vi "界面UI.vi"() -> ()   [LabVIEW 2016, in "德润超标留样.lvlib"]
uses:
  <vilib>/Utility/miscctls.llb/LVPointTypeDef.ctl
  <vilib>/Utility/config.llb/NI_LVConfig.lvlib
panel:
  in  "时间等比采样":u16=10
  in  "单次采样量":u16=500
  in  "修改门禁密码":bool
  in  "远程复位":bool
  in  "排空当前瓶":bool
  in  "采样方式":enum16{"单采", "双重"}(ring)
  in  "远程留样":bool
  in  "选择留样瓶":bool
  in  "排空留样瓶":bool
  out "采样器状态":T1
  out "Registers":u16[](array[numeric])
  in  "打开串口":bool
  in  "释放串口":bool
  in  "留样模式":T2(ring)=enum."外控留样"
  in  "采样启动":bool
  in  "停止命令":bool
  in  "切换采样器状态":bool
  in  "时间校准":bool
  out "source":string
  out "通讯":bool
  # "只在待机时启动有效"
  # "只在停止时切换有效"
  # "只在待机时启动有效"
  # "只在待机时切换有效"
  # "只在待机时启动有效"
  # "默认：500ml（5-1000）ml （只在停止时写有效）"
  # "默认：10min（2-9999）min （只在停止时写有效）"
  # "德润DR803L超标留样"
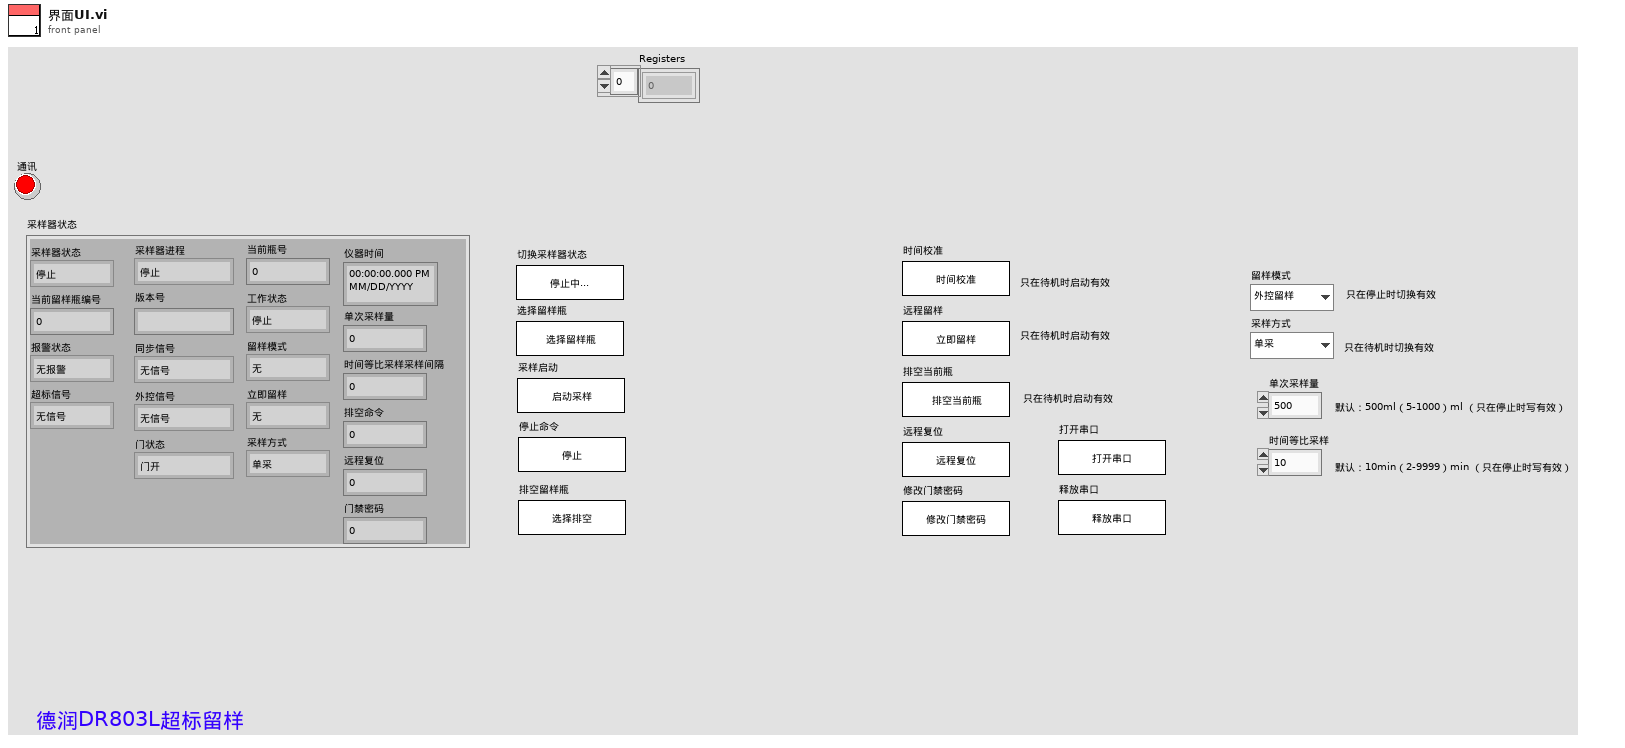
[diagram p1: front panel]
types:
  T1 = cluster{"采样器状态":enum16{"停止", "运行"}, "当前留样瓶编号":u16, "报警状态":enum16{"无报警", "缺水报警"}, "超标信号":enum16{"无信号", "超标信号"}, "采样器进程":enum16{"停止", "待机", "定位校正", "移除瓶盖", "采样瓶排空", "管路润洗", "管存", "进样", "瓶盖密封", "管路排空", "调整采样位置", "采样结束", "采样瓶润洗", "瓶润洗排空"}, "版本号":string, "同步信号":enum16{"无信号", "同步信号"}, "外控信号":enum16{"无信号", "外控信号"}, "门状态":enum16{"门开", "门关"}, "当前瓶号":u16, "工作状态":enum16{"停止", "采样中"}, "留样模式":enum16{"无", "定时留样", "时间等比例", "超标留样", "同步留样", "外控留样"}, "立即留样":enum16{"无", "远程留样"}, "采样方式":enum16{"单采", "双重"}, "仪器时间":timestamp, "单次采样量":u16, "时间等比采样采样间隔":u16, "排空命令":u16, "远程复位":u16, "门禁密码":u16}
  T2 = enum16{"", "定时留样", "时间等比", "超标留样", "同步留样", "外控留样"}
  T3 = typedef "LVPointTypeDef.ctl" = cluster{"Horizontal":i16, "Vertical":i16}
  T4 = typedef "NI_LVConfig.lvlib/Config Data RefNum.ctl" = refnum<k1>
  T5 = typedef "LVDateTimeRec.ctl" = cluster{"秒数的小数部分":dbl, "秒":i32, "分":i32, "时":i32, "日":i32, "月":i32, "年":i32, "天数（周）":i32, "天数（年）":i32, "DST":i32}
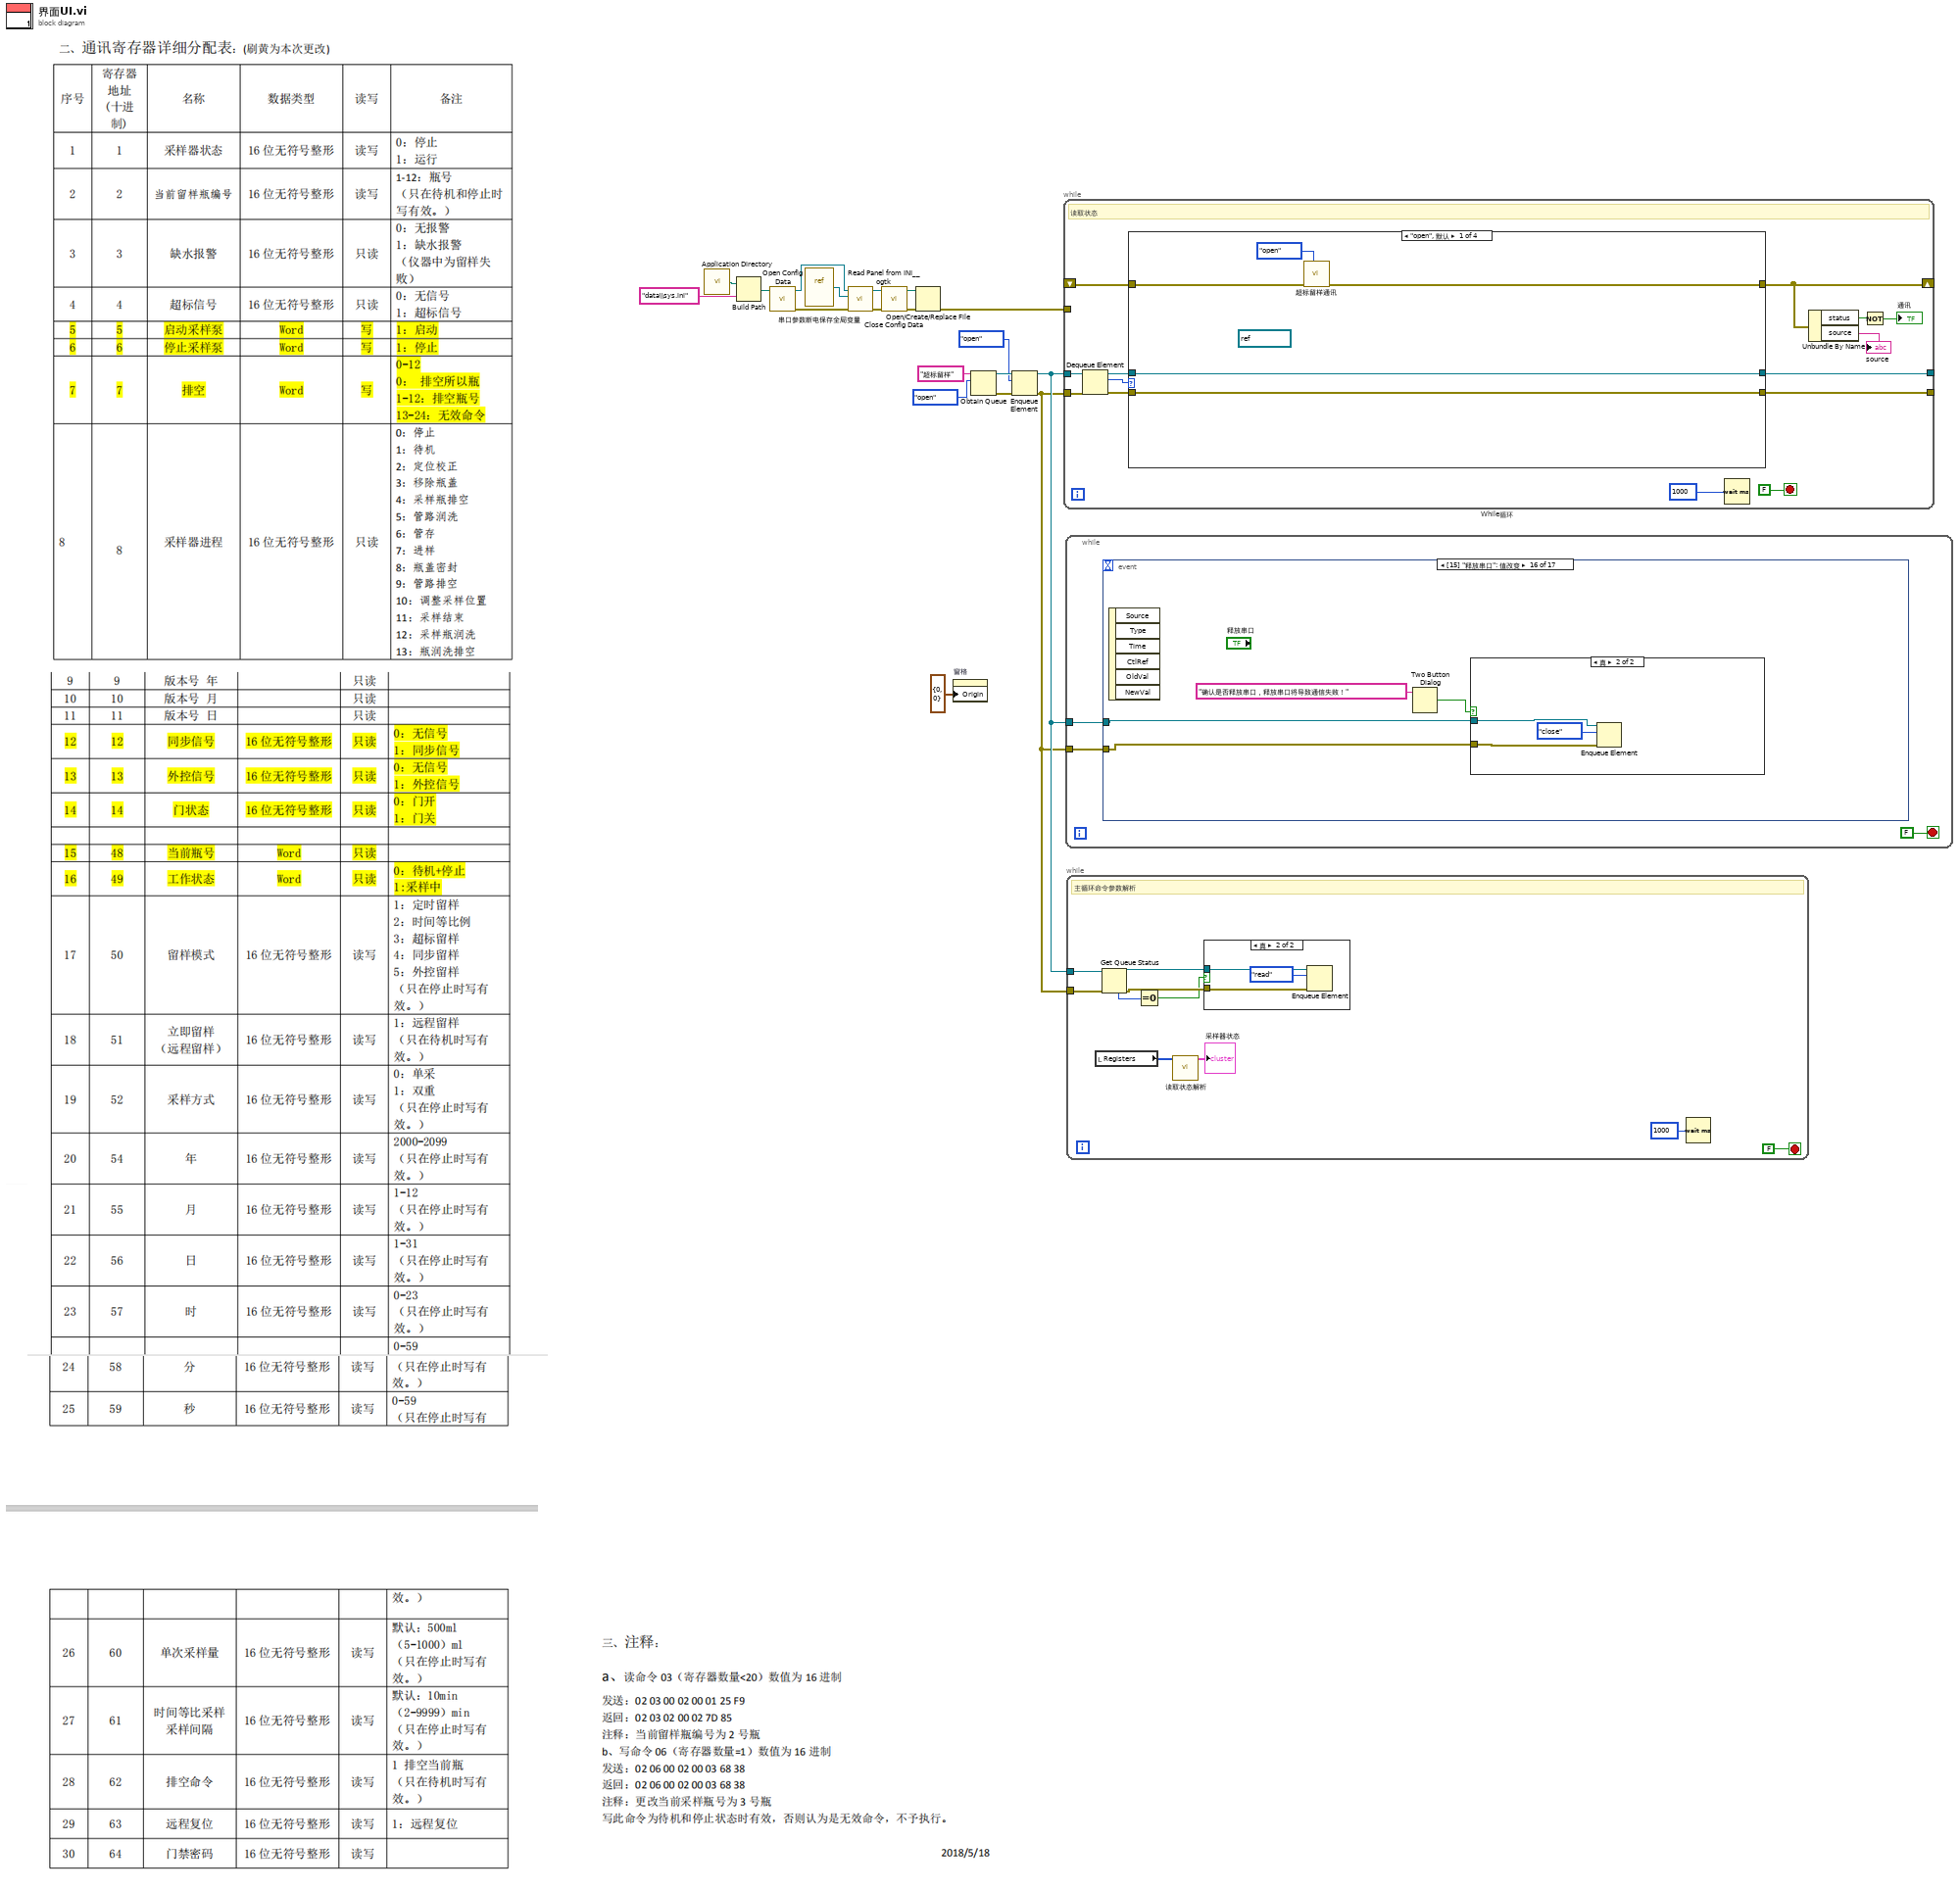
[diagram p0: block diagram]
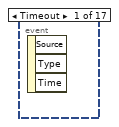
[diagram p2: hidden frame]
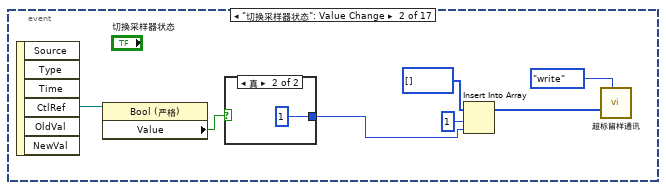
[diagram p3: hidden frame]
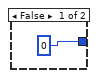
[diagram p4: hidden frame]
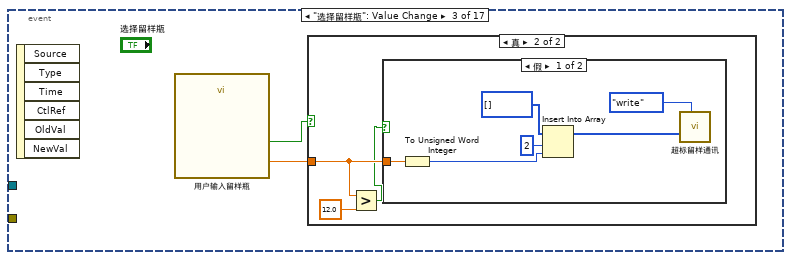
[diagram p5: hidden frame]
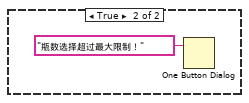
[diagram p7: hidden frame]
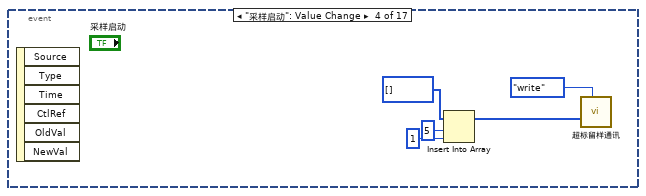
[diagram p8: hidden frame]
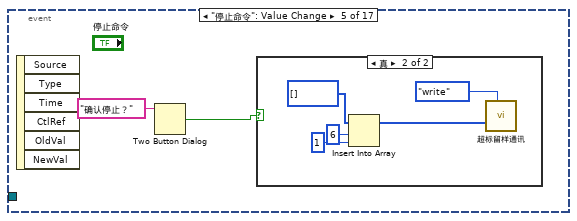
[diagram p9: hidden frame]
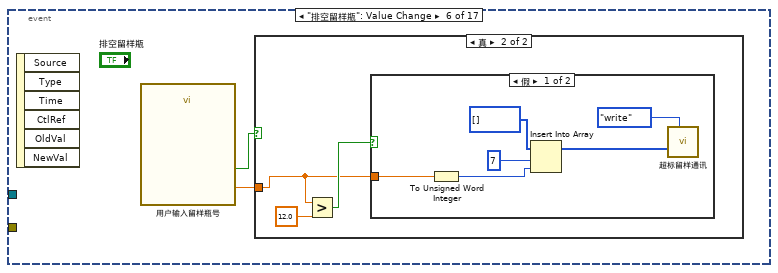
[diagram p11: hidden frame]
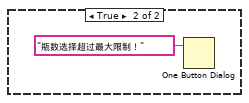
[diagram p13: hidden frame]
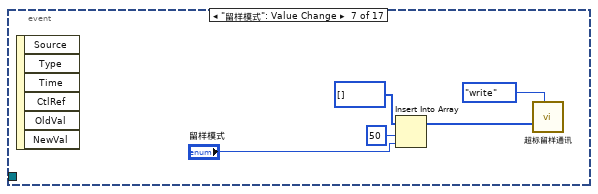
[diagram p14: hidden frame]
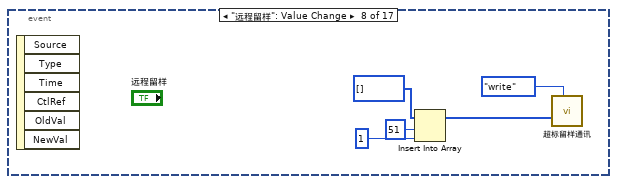
[diagram p15: hidden frame]
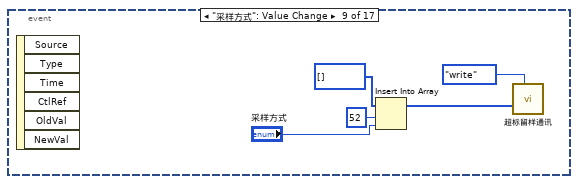
[diagram p16: hidden frame]
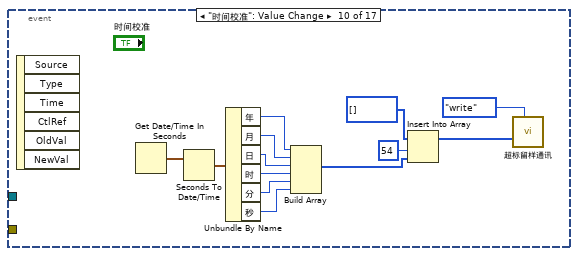
[diagram p17: hidden frame]
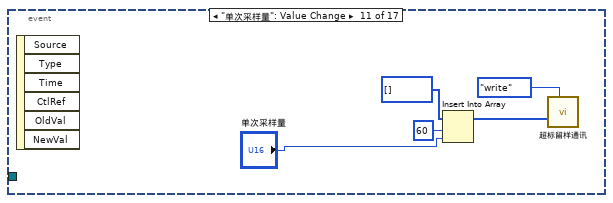
[diagram p18: hidden frame]
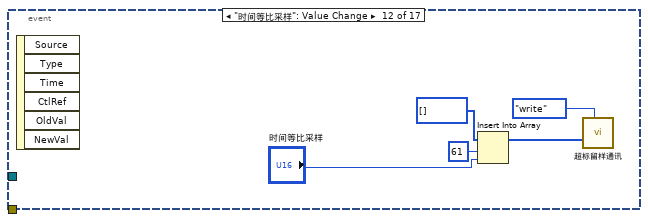
[diagram p19: hidden frame]
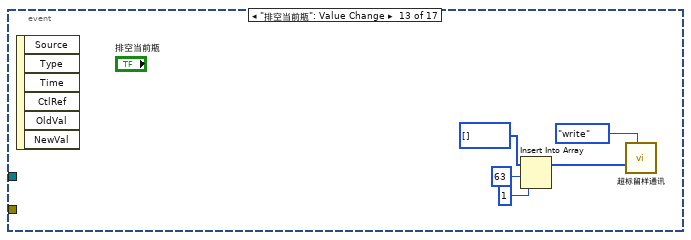
[diagram p20: hidden frame]
diagram:
  n1 = call <vilib>:"Application Directory.vi"() -> ("Application Directory"=w11:path)
  n2 = Build Path(base path=w11, name or relative path="data\\sys.ini" ("名称或相对路径")) -> (appended path=w9:path)
  n3 = call <vilib>:"Open Config Data.vi"("configuration file path"=w9) -> ("error out"=w5:errorcluster, "refnum"=w8:T4)  [unwired: 8 in, 1 out]
  n4 = vi-ref "串口参数断电保存全局变量.vi"() -> (w7:refnum<vi>)
  n5 = call <userlib>:"Read Panel from INI__ogtk.vi"("error in (no error)"=w5, "VI ref"=w7, "refnum"=w8) -> ("error out"=w4:errorcluster, "refnum out"=w6:T4)  [unwired: 7 in]
  n6 = call <vilib>:"Close Config Data.vi"("error in (no error)"=w4, "refnum"=w6) -> ("error out"=w3:errorcluster, "file path"=w2:path)  [unwired: 8 in]
  n7 = Open/Create/Replace File(file path (use dialog)=w2, error in=w3) -> (error out=w1:errorcluster)  [unwired: 4 in, 2 out]
  n8 = property on="窗格" class="Pane"("Origin"=T3 {"Horizontal"=0, "Vertical"=0} ("原点")) -> ()  [unwired: 2 in, 2 out]
  n9 = Obtain Queue(name (unnamed)="超标留样" ("名称（未命名）"), element data type=enum16{"open", "read", "write", "close"}."open") -> (queue out=w17:refnum<queue>, error out=w16:errorcluster)  [unwired: 3 in, 1 out]
  n10 = Enqueue Element(queue=w17, element=enum16{"open", "read", "write", "close"}."open", error in (no error)=w16) -> (queue out=w14:refnum<queue>, error out=w13:errorcluster)  [unwired: 1 in, 1 out]
  n11 = while "While循环" {
    tunnel: w14 -> [w31]
    tunnel: w13 -> [w30]
    tunnel: [w26] -> _
    tunnel: [w25] -> _
    shift-right: [w20] -> _
    shift-left: _ -> [w24]
    tunnel: w1 -> [_]
    stop <- FALSE stop-if-true
    # "读取状态"
    n12 = Dequeue Element(queue=w31, error in (no error)=w30) -> (queue out=w28:refnum<queue>, element=w29:enum16{"open", "read", "write", "close"}, error out=w27:errorcluster)  [unwired: 1 in, 1 out]
    n13 = case shown="\"open\", 默认" w29 {
      tunnel: [w38 w40 w51 w56] -> w20
      tunnel: w28 -> [w37 w45 w50 w54]
      tunnel: w27 -> [w36 w44 w49 w53]
      tunnel: [w37 w45 w50 w54] -> w26
      tunnel: [w36 w44 w49 w53] -> w25
      tunnel: w24 -> [w34 w46 w52 w57]
      frame "open", Default {
        (unwired) refnum<visa-resource-name> "COM2" ("VISA resource name")
        n14 = call "超标留样通讯.vi"("STEP"=enum16{"open", "read", "write", "close"}."open", "Error in"=w34) -> ("error out"=w38:errorcluster)  [unwired: 6 in, 3 out]
      }
      frame "read" {
        n15 = call "超标留样通讯.vi"("STEP"=enum16{"open", "read", "write", "close"}."read", "Error in"=w46, "quantity"=u16 70, "starting address"=u16 0) -> ("error out"=w40:errorcluster, "Registers"=w39:u16[])  [unwired: 4 in, 2 out]
        n16 = case shown="无错误" w40 {
          tunnel: w39 -> [w47 _]
          frame No Error {
            "Registers" <- w47
          }
          frame Error {
          }
        }
      }
      frame "write" {
        n17 = call "超标留样通讯.vi"("STEP"=enum16{"open", "read", "write", "close"}."write", "Error in"=w52) -> ("error out"=w51:errorcluster)  [unwired: 6 in, 3 out]
      }
      frame "close" {
        n18 = call "超标留样通讯.vi"("STEP"=enum16{"open", "read", "write", "close"}."close", "Error in"=w57) -> ("error out"=w56:errorcluster)  [unwired: 6 in, 3 out]
      }
    }
    n19 = Wait (ms)(milliseconds to wait=u32 1000 ("等待时间（毫秒）")) -> ()  [unwired: 1 out]
    n20 = Unbundle By Name(w20) -> ("status"=w21:bool, "source"=→"source":string)
    n21 = Not(x=w21) -> (.not. x?=→"通讯":bool)
  }
  n22 = while {
    tunnel: w14 -> [w59]
    tunnel: w13 -> [w58]
    stop <- FALSE stop-if-true
    n23 = event shown="[15] \"释放串口\": 值改变" {
      selector: _ -> [_ _ _ _ _ _ _ _ _ _ _ _ _ _ _ _ _]
      dyn-events: _ -> [_ _ _ _ _ _ _ _ _ _ _ _ _ _ _ _ _]
      timeout: _ -> [_ _ _ _ _ _ _ _ _ _ _ _ _ _ _ _ _]
      tunnel: w59 -> [_ _ _ _ _ _ _ _ _ _ _ _ _ _ _ w168 w174]
      tunnel: w58 -> [_ _ _ _ _ _ _ _ _ _ _ _ _ _ _ w167 w173]
      event Timeout {
        n24 = event-data() -> ()  [unwired: 1 in, 3 out]
      }
      event "切换采样器状态": Value Change {
        n25 = event-data() -> ("CtlRef"=w66:refnum<vi>)  [unwired: 1 in, 5 out]
        n26 = property class="Bool (严格)"(reference=w66) -> ("Value"=w63:bool)  [unwired: 1 in, 2 out]
        n27 = case shown="真" w63 {
          tunnel: [u16 0 ("索引") u16 1 ("索引")] -> w62
          frame False {
          }
          frame True {
          }
        }
        n28 = Insert Into Array(array=u16[] [] ("values"), index=1 ("索引"), new element=w62) -> (w61:u16[])
        n29 = call "超标留样通讯.vi"("STEP"=enum16{"open", "read", "write", "close"}."write", "values"=w61) -> ()  [unwired: 6 in, 4 out]
      }
      event "选择留样瓶": Value Change {
        n30 = event-data() -> ()  [unwired: 1 in, 6 out]
        n31 = call "用户输入留样瓶"() -> ("留样瓶1~12"=w71:dbl, "确定"=w70:bool)  [unwired: 17 in, 1 out]
        n32 = case shown="真" w70 {
          tunnel: w71 -> [_ w73]
          frame False {
          }
          frame True {
            n33 = Greater?(x=w73, y=12.0) -> (0:w72:bool)
            n34 = case shown="假" w72 {
              tunnel: w73 -> [w80 _]
              frame False {
                n35 = To Unsigned Word Integer(number=w80) -> (unsigned 16bit integer=w75:u16)
                n36 = Insert Into Array(array=u16[] [] ("values"), index=2 ("索引"), new element=w75) -> (w76:u16[])
                n37 = call "超标留样通讯.vi"("STEP"=enum16{"open", "read", "write", "close"}."write", "values"=w76) -> ()  [unwired: 6 in, 4 out]
              }
              frame True {
                n38 = One Button Dialog(message="瓶数选择超过最大限制！" ("消息")) -> ()  [unwired: 1 in, 1 out]
              }
            }
          }
        }
      }
      event "采样启动": Value Change {
        n39 = event-data() -> ()  [unwired: 1 in, 6 out]
        n40 = Insert Into Array(array=u16[] [] ("values"), index=5 ("索引"), new element=u16 1 ("新元素/子数组")) -> (w83:u16[])
        n41 = call "超标留样通讯.vi"("STEP"=enum16{"open", "read", "write", "close"}."write", "values"=w83) -> ()  [unwired: 6 in, 4 out]
      }
      event "停止命令": Value Change {
        n42 = event-data() -> ()  [unwired: 1 in, 6 out]
        n43 = Two Button Dialog(message="确认停止？" ("消息")) -> (T button?=w87:bool)  [unwired: 2 in]
        n44 = case shown="真" w87 {
          frame False {
          }
          frame True {
            n45 = Insert Into Array(array=u16[] [] ("values"), index=6 ("索引"), new element=u16 1 ("新元素/子数组")) -> (w90:u16[])
            n46 = call "超标留样通讯.vi"("STEP"=enum16{"open", "read", "write", "close"}."write", "values"=w90) -> ()  [unwired: 6 in, 4 out]
          }
        }
      }
      event "排空留样瓶": Value Change {
        n47 = event-data() -> ()  [unwired: 1 in, 6 out]
        n48 = call "用户输入留样瓶号"() -> ("0~12(0:排空所有瓶,1-12:排空瓶号)"=w95:dbl, "确定"=w94:bool)  [unwired: 17 in, 1 out]
        n49 = case shown="真" w94 {
          tunnel: w95 -> [_ w96]
          frame False {
          }
          frame True {
            n50 = Greater?(x=w96, y=12.0) -> (0:w97:bool)
            n51 = case shown="假" w97 {
              tunnel: w96 -> [w104 _]
              frame False {
                n52 = To Unsigned Word Integer(number=w104) -> (unsigned 16bit integer=w99:u16)
                n53 = Insert Into Array(array=u16[] [] ("values"), index=7 ("索引"), new element=w99) -> (w100:u16[])
                n54 = call "超标留样通讯.vi"("STEP"=enum16{"open", "read", "write", "close"}."write", "values"=w100) -> ()  [unwired: 6 in, 4 out]
              }
              frame True {
                n55 = One Button Dialog(message="瓶数选择超过最大限制！" ("消息")) -> ()  [unwired: 1 in, 1 out]
              }
            }
          }
        }
      }
      event "留样模式": Value Change {
        n56 = event-data() -> ()  [unwired: 1 in, 6 out]
        n57 = Insert Into Array(array=u16[] [] ("values"), index=50 ("索引"), new element="留样模式") -> (w107:u16[])
        n58 = call "超标留样通讯.vi"("STEP"=enum16{"open", "read", "write", "close"}."write", "values"=w107) -> ()  [unwired: 6 in, 4 out]
      }
      event "远程留样": Value Change {
        n59 = event-data() -> ()  [unwired: 1 in, 6 out]
        n60 = Insert Into Array(array=u16[] [] ("values"), index=51 ("索引"), new element=u16 1 ("新元素/子数组")) -> (w112:u16[])
        n61 = call "超标留样通讯.vi"("STEP"=enum16{"open", "read", "write", "close"}."write", "values"=w112) -> ()  [unwired: 6 in, 4 out]
      }
      event "采样方式": Value Change {
        n62 = event-data() -> ()  [unwired: 1 in, 6 out]
        n63 = Insert Into Array(array=u16[] [] ("values"), index=52 ("索引"), new element="采样方式") -> (w117:u16[])
        n64 = call "超标留样通讯.vi"("STEP"=enum16{"open", "read", "write", "close"}."write", "values"=w117) -> ()  [unwired: 6 in, 4 out]
      }
      event "时间校准": Value Change {
        n65 = event-data() -> ()  [unwired: 1 in, 6 out]
        n66 = Get Date/Time In Seconds() -> (seconds since 1Jan1904=w133:timestamp)
        n67 = Seconds To Date/Time(time stamp (now)=w133) -> (date time rec=w132:T5)  [unwired: 1 in]
        n68 = Unbundle By Name(w132) -> ("年"=w127:i32, "月"=w126:i32, "日"=w125:i32, "时"=w124:i32, "分"=w123:i32, "秒"=w122:i32)
        n69 = Build Array(w127, w126, w125, w124, w123, w122) -> (w121:i32[])
        n70 = Insert Into Array(array=u16[] [] ("values"), index=54 ("索引"), new element=w121) -> (w128:u16[])
        n71 = call "超标留样通讯.vi"("STEP"=enum16{"open", "read", "write", "close"}."write", "values"=w128) -> ()  [unwired: 6 in, 4 out]
      }
      event "单次采样量": Value Change {
        n72 = event-data() -> ()  [unwired: 1 in, 6 out]
        n73 = Insert Into Array(array=u16[] [] ("values"), index=60 ("索引"), new element="单次采样量") -> (w135:u16[])
        n74 = call "超标留样通讯.vi"("STEP"=enum16{"open", "read", "write", "close"}."write", "values"=w135) -> ()  [unwired: 6 in, 4 out]
      }
      event "时间等比采样": Value Change {
        n75 = event-data() -> ()  [unwired: 1 in, 6 out]
        n76 = Insert Into Array(array=u16[] [] ("values"), index=61 ("索引"), new element="时间等比采样") -> (w140:u16[])
        n77 = call "超标留样通讯.vi"("STEP"=enum16{"open", "read", "write", "close"}."write", "values"=w140) -> ()  [unwired: 6 in, 4 out]
      }
      event "排空当前瓶": Value Change {
        n78 = event-data() -> ()  [unwired: 1 in, 6 out]
        n79 = Insert Into Array(array=u16[] [] ("values"), index=63 ("索引"), new element=u16 1 ("新元素/子数组")) -> (w145:u16[])
        n80 = call "超标留样通讯.vi"("STEP"=enum16{"open", "read", "write", "close"}."write", "values"=w145) -> ()  [unwired: 6 in, 4 out]
      }
      event "远程复位": Value Change {
        n81 = event-data() -> ()  [unwired: 1 in, 6 out]
        n82 = Insert Into Array(array=u16[] [] ("values"), index=64 ("索引"), new element=u16 1 ("新元素/子数组")) -> (w150:u16[])
        n83 = call "超标留样通讯.vi"("STEP"=enum16{"open", "read", "write", "close"}."write", "values"=w150) -> ()  [unwired: 6 in, 4 out]
      }
      event "修改门禁密码": Value Change {
        n84 = event-data() -> ()  [unwired: 1 in, 6 out]
        n85 = Two Button Dialog(message="确定修改门禁密码？" ("消息")) -> (T button?=w154:bool)  [unwired: 2 in]
        n86 = case shown="真" w154 {
          frame False {
          }
          frame True {
            n87 = call "数字键盘.vi"("OldNumber"=sgl 123456.0) -> ("NewNumber"=w158:sgl)
            n88 = Less?(x=w158, y=sgl 65535.0) -> (x < y?=w156:bool)
            n89 = case shown="真" w156 {
              tunnel: w158 -> [_ w161]
              frame False {
              }
              frame True {
                n90 = To Unsigned Word Integer(number=w161) -> (unsigned 16bit integer=w160:u16)
                n91 = Insert Into Array(array=u16[] [] ("values"), index=65 ("索引"), new element=w160) -> (w162:u16[])
                n92 = call "超标留样通讯.vi"("STEP"=enum16{"open", "read", "write", "close"}."write", "values"=w162) -> ()  [unwired: 6 in, 4 out]
              }
            }
          }
        }
      }
      event "释放串口": Value Change {
        n93 = event-data() -> ()  [unwired: 1 in, 6 out]
        n94 = Two Button Dialog(message="确认是否释放串口，释放串口将导致通信失败！" ("消息")) -> (T button?=w166:bool)  [unwired: 2 in]
        n95 = case shown="真" w166 {
          tunnel: w168 -> [_ w171]
          tunnel: w167 -> [_ w170]
          frame False {
          }
          frame True {
            n96 = Enqueue Element(queue=w171, element=enum16{"open", "read", "write", "close"}."close" ("元素"), error in (no error)=w170) -> ()  [unwired: 1 in, 3 out]
          }
        }
      }
      event "打开串口": Value Change {
        n97 = event-data() -> ()  [unwired: 1 in, 6 out]
        n98 = global read "串口参数断电保存全局变量.vi" "VISA resource name"() -> (w182:refnum<visa-resource-name>)
        n99 = global read "串口参数断电保存全局变量.vi" "MB通信方式选择"() -> (w183:enum16{"串口", "TCP"})
        n100 = global read "串口参数断电保存全局变量.vi" "PORT"() -> (w180:string)
        n101 = global read "串口参数断电保存全局变量.vi" "IP"() -> (w181:string)
        n102 = call "串口配置.vi"("PORT"=w180, "IP"=w181, "MB通信方式选择"=w183, "请选择串口:"=w182) -> ("PORT 2"=w176:string, "IP 2"=w177:string, "确认 2"=w179:bool, "VISA资源名称 2"=w178:refnum<visa-resource-name>, "MB通信方式选择 2"=w175:enum16{"串口", "TCP"})  [unwired: 3 in]
        n103 = case shown="真" w179 {
          tunnel: w178 -> [_ w191]
          tunnel: w177 -> [_ w190]
          tunnel: w176 -> [_ w189]
          tunnel: w175 -> [_ w188]
          tunnel: w174 -> [_ w187]
          tunnel: w173 -> [_ w185]
          frame False {
          }
          frame True {
            n104 = flat-sequence {
              tunnel: w191 -> [w197]
              tunnel: w190 -> [w196]
              tunnel: w189 -> [w195]
              tunnel: w188 -> [w194]
              tunnel: w187 -> [w193]
              tunnel: [w193] -> w186
              tunnel: w185 -> [w192]
              tunnel: [w192] -> w184
              tunnel: w186 -> [w199]
              tunnel: w184 -> [w198]
              frame #0 {
                n105 = global write "串口参数断电保存全局变量.vi" "VISA resource name"(w197) -> ()
                n106 = global write "串口参数断电保存全局变量.vi" "MB通信方式选择"(w194) -> ()
                n107 = global write "串口参数断电保存全局变量.vi" "PORT"(w195) -> ()
                n108 = global write "串口参数断电保存全局变量.vi" "IP"(w196) -> ()
              }
              frame #1 {
                n109 = call <vilib>:"Application Directory.vi"() -> ("Application Directory"=w202:path)
                n110 = Build Path(base path=w202, name or relative path="data\\sys.ini" ("名称或相对路径")) -> (appended path=w203:path)
                n111 = Enqueue Element(queue=w199, element=enum16{"open", "read", "write", "close"}."open" ("元素"), error in (no error)=w198) -> ()  [unwired: 1 in, 3 out]
                n112 = call <vilib>:"Open Config Data.vi"("configuration file path"=w203) -> ("error out"=w207:errorcluster, "refnum"=w204:T4)  [unwired: 8 in, 1 out]
                n113 = vi-ref "斯坦道CODMn.lvlib:CODMn断电保存全局变量.vi"() -> (w205:refnum<vi>)
                n114 = call <userlib>:"Write Panel to INI__ogtk.vi"("error in (no error)"=w207, "VI ref"=w205, "refnum"=w204) -> ("error out"=w208:errorcluster, "refnum out"=w206:T4)  [unwired: 7 in]
                n115 = call <vilib>:"Close Config Data.vi"("error in (no error)"=w208, "refnum"=w206) -> ("error out"=w213:errorcluster, "file path"=w214:path)  [unwired: 8 in]
                n116 = Open/Create/Replace File(file path (use dialog)=w214, error in=w213) -> (refnum out=w210:refnum<file>, error out=w209:errorcluster)  [unwired: 4 in, 1 out]
                n117 = Flush File(refnum=w210, error in=w209) -> (refnum out=w211:refnum<file>, error out=w212:errorcluster)
                n118 = Close File(refnum=w211, error in=w212) -> ()  [unwired: 2 out]
              }
            }
          }
        }
      }
    }
  }
  n119 = while {
    tunnel: w14 -> [w222]
    tunnel: w13 -> [w221]
    stop <- FALSE stop-if-true
    # "主循环命令参数解析"
    n120 = local read "Registers"() -> (w216:u16[])
    n121 = Get Queue Status(queue=w222, error in (no error)=w221) -> (queue out=w219:refnum<queue>, error out=w218:errorcluster, # elements in queue=w220:i32)  [unwired: 1 in, 5 out]
    n122 = Equal To 0?(x=w220) -> (x = 0?=w217:bool)
    n123 = call "读取状态解析.vi"("Registers"=w216) -> ("采样器状态"=→"采样器状态":T1)  [unwired: 9 in, 1 out]
    n124 = case shown="真" w217 {
      tunnel: w219 -> [_ w226]
      tunnel: w218 -> [_ w225]
      frame False {
      }
      frame True {
        n125 = Enqueue Element(queue=w226, element=enum16{"open", "read", "write", "close"}."read" ("元素"), error in (no error)=w225) -> ()  [unwired: 1 in, 3 out]
      }
    }
    n126 = Wait (ms)(milliseconds to wait=u32 1000 ("等待时间（毫秒）")) -> ()  [unwired: 1 out]
  }
